vi "Track movement.vi"(8 "error in (no error)":errorcluster, 10 "tracking code":string, 11 "Motor in":refnum<class "Motor.lvclass">) -> (0 "error out":errorcluster, 1 "error":bool, 2 "moving":bool, 3 "Motor out":refnum<class "Motor.lvclass">)   [LabVIEW 2018, in "Motor.lvclass"]
uses:
  Motor.lvclass
  Motor.lvclass/Motor.ctl
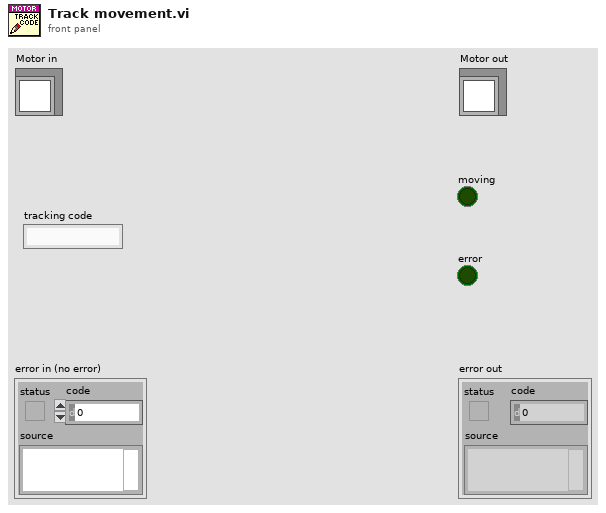
[diagram p1: front panel]
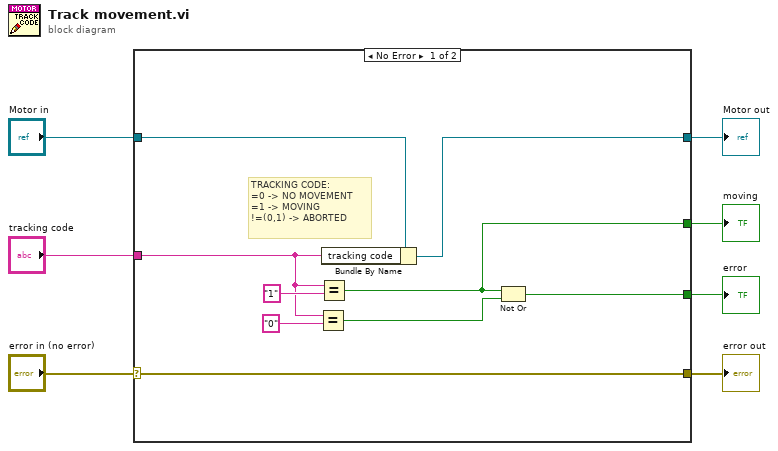
[diagram p0: block diagram]
diagram:
  n1 = case shown="No Error" "error in (no error)" {
    selector: "error in (no error)" -> [w15 w17]
    tunnel: [w15 w17] -> w6
    tunnel: [w14 w18] -> w4
    tunnel: "Motor in" -> [w16 w18]
    tunnel: "tracking code" -> [w11 _]
    tunnel: [w9 _] -> w2
    tunnel: [w8 _] -> w1
    frame No Error {
      # "TRACKING CODE:\n=0 -> NO MOVEMENT\n=1 -> MOVING\n!=(0,1) -> ABORTED"
      n2 = Equal?(x=w11, y="0") -> (x = y?=w10:bool)
      n3 = Equal?(x=w11, y="1") -> (x = y?=w9:bool)
      n4 = Bundle By Name(cluster=w16, "tracking code"=w11) -> (w14:refnum<class "Motor.lvclass">)
      n5 = Not Or(1:w10, 2:w9) -> (0:w8:bool)
    }
    frame Error {
    }
  }
  "error out" <- w6
  "Motor out" <- w4
  "moving" <- w2
  "error" <- w1
